vi "Simple Child Node Sending.vi"(4 "Priority":i32, 5 "Emergency Send?":bool, 7 "Node Actor In":refnum<class "Node Actor.lvclass">, 10 "Message In":refnum<class "Message.lvclass">, 11 "ID In":i64) -> ()   [LabVIEW 2024]
uses:
  Ancestor Class/Message/Message.lvclass
  Ancestor Class/Actor/Node Actor/Node Actor.lvclass
  C:/Users/iio/Desktop/Bussiness/Tricorn Re/Madelbrot 4.0/General Library/Ancestor Class/Actor/Root Actor/Root Actor.lvclass
  C:/Users/iio/Desktop/Bussiness/Tricorn Re/Madelbrot 4.0/General Library/Ancestor Class/Actor/System Actor/System Actor.lvclass
  Ancestor Class/Actor/Root Actor/Root Actor.lvclass/Root Actor.ctl
  Ancestor Class/Actor/System Actor/System Actor.lvclass/System Actor.ctl
  Ancestor Class/Message/Message.lvclass/Message.ctl
  Ancestor Class/Actor/Node Actor/Public Data/Read Static Child Messenger.vi
  Ancestor Class/Actor/System Actor/Public Data/Read ID.vi
  Ancestor Class/Message/Write Sender ID.vi
  Ancestor Class/Actor/Root Actor/Protected Data/Read Static System Messenger.vi
  Ancestor Class/Messenger/Messenger/Messenger.lvclass
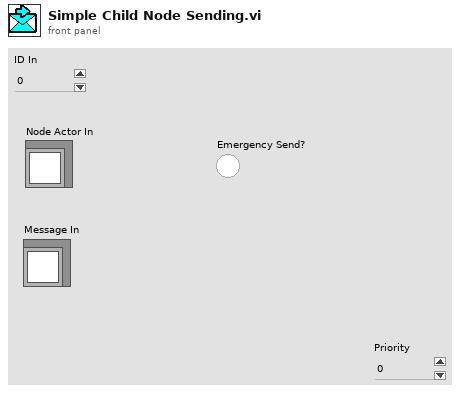
[diagram p1: front panel]
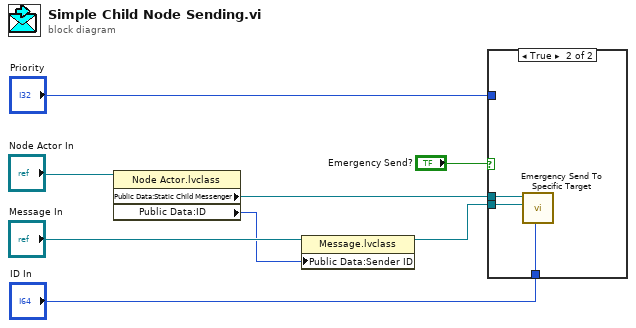
[diagram p0: block diagram]
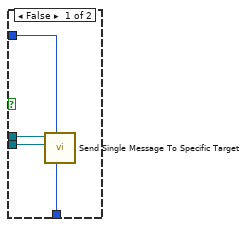
[diagram p2: hidden frame]
diagram:
  n1 = property class="Node Actor.lvclass"(reference="Node Actor In") -> ("Public Data:Static Child Messenger"=w8:refnum<class "Messenger.lvclass">, "Public Data:ID"=w2:i64)  [unwired: 1 in, 2 out]
  n2 = property class="Message.lvclass"(reference="Message In", "Public Data:Sender ID"=w2) -> (reference out=w3:refnum<class "Message.lvclass">)  [unwired: 1 in, 1 out]
  n3 = case shown="True" "Emergency Send?" {
    tunnel: w3 -> [w12 w14]
    tunnel: w8 -> [w11 w15]
    tunnel: "Priority" -> [w10 _]
    tunnel: "ID In" -> [w9 w13]
    frame False {
      n4 = call-dynamic "Send Single Message To Specific Target.vi"("Paras In"=w9, "Priority"=w10, "Message In"=w12, "Messenger in"=w11) -> ()  [unwired: 6 in, 2 out]
    }
    frame True {
      n5 = call-dynamic "Emergency Send To Specific Target.vi"("Paras In"=w13, "Message In"=w14, "Messenger in"=w15) -> ()  [unwired: 7 in, 2 out]
    }
  }
